vi "Lcalc.vi"(4 "A - B":T1) -> (0 "l3":dbl, 1 "l2":dbl, 2 "l1":dbl)   [LabVIEW 2019]
uses:
  <vilib>/Analysis/Matrix/Datatypes/RealMatrix.ctl
  <vilib>/Analysis/_algsub.llb/Real Vector Norm.vi
  <vilib>/Analysis/NI_AALPro.lvlib
  <vilib>/Analysis/Matrix/NI_Matrix.lvlib
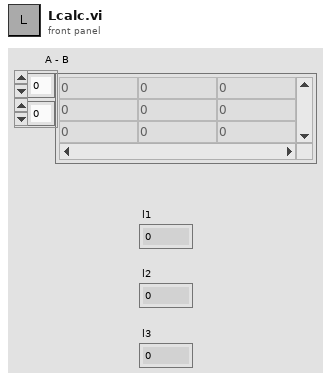
[diagram p1: front panel]
types:
  T1 = typedef "NI_Matrix.lvlib/RealMatrix.ctl" = dbl[][]
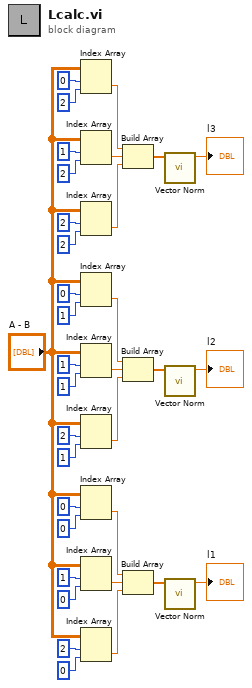
[diagram p0: block diagram]
diagram:
  n1 = Index Array(array="A - B", index (row)=0, index (col)=2) -> (element=w8:dbl)
  n2 = Index Array(array="A - B", index (row)=1, index (col)=2) -> (element=w6:dbl)
  n3 = Index Array(array="A - B", index (row)=2, index (col)=2) -> (element=w7:dbl)
  n4 = Index Array(array="A - B", index (row)=0, index (col)=1) -> (element=w17:dbl)
  n5 = Index Array(array="A - B", index (row)=1, index (col)=1) -> (element=w16:dbl)
  n6 = Index Array(array="A - B", index (row)=2, index (col)=1) -> (element=w15:dbl)
  n7 = Index Array(array="A - B", index (row)=0, index (col)=0) -> (element=w31:dbl)
  n8 = Index Array(array="A - B", index (row)=1, index (col)=0) -> (element=w26:dbl)
  n9 = Index Array(array="A - B", index (row)=2, index (col)=0) -> (element=w25:dbl)
  n10 = Build Array(w8, w6, w7) -> (w2:dbl[])
  n11 = Build Array(w17, w16, w15) -> (w3:dbl[])
  n12 = Build Array(w31, w26, w25) -> (w24:dbl[])
  n13 = call-poly <vilib>:"Vector Norm.vi"("Input Vector"=w2) -> ("norm"=→"l3":dbl)  [unwired: 9 in, 1 out]
  n14 = call-poly <vilib>:"Vector Norm.vi"("Input Vector"=w3) -> ("norm"=→"l2":dbl)  [unwired: 9 in, 1 out]
  n15 = call-poly <vilib>:"Vector Norm.vi"("Input Vector"=w24) -> ("norm"=→"l1":dbl)  [unwired: 9 in, 1 out]
